vi "PublishConnected.vi"(8 "error in (no error)":errorcluster, 10 "Connected":bool=TRUE, 11 "TCPComEvents in":refnum<class "TCPComEvents.lvclass">) -> (0 "error out":errorcluster, 3 "TCPComEvents out":refnum<class "TCPComEvents.lvclass">)   [LabVIEW 2016, in "TCPComEvents.lvclass"]
uses:
  TCPComEvents.lvclass
  TCPComEvents.lvclass/TCPComEvents.ctl
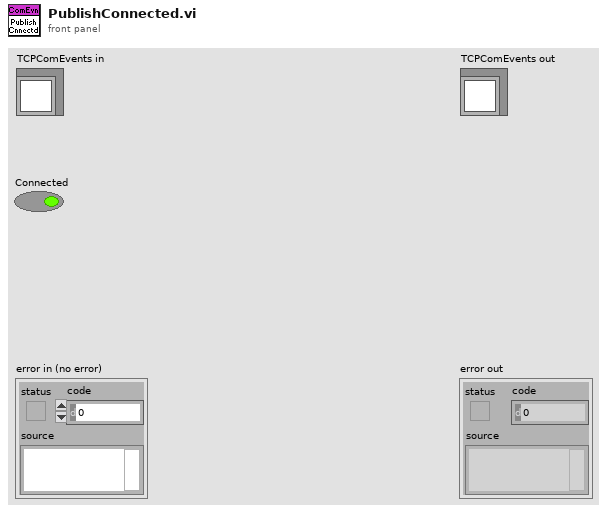
[diagram p1: front panel]
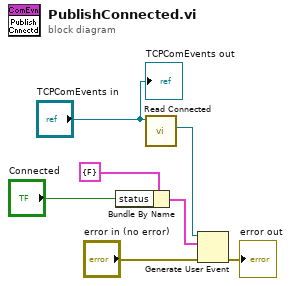
[diagram p0: block diagram]
diagram:
  n1 = Bundle By Name(cluster=cluster{"status":bool} {"status"=FALSE} ("event data"), "status"="Connected") -> (w1:cluster{"status":bool})
  n2 = call "Read Connected.vi"("TCPComEvents in"="TCPComEvents in") -> ("Connected"=w6:refnum<user-event>)  [unwired: 8 in, 2 out]
  n3 = Generate User Event(user event=w6, event data cluster=w1, error in="error in (no error)") -> (error out=→"error out":errorcluster)  [unwired: 1 in, 1 out]
  "TCPComEvents out" <- "TCPComEvents in"
